vi "CheckRunProbe.vi"(0 "UiDefinition":T1) -> ()   [LabVIEW 2020]
uses:
  UIReferences.ctl
  C:/Users/User/Desktop/Automation/CurrentVersion/LabviewDXFViewer/bin/Release/LabviewDXFViewer.exe
  LabviewDXFViewer/bin/Release/LabviewDXFViewer.exe
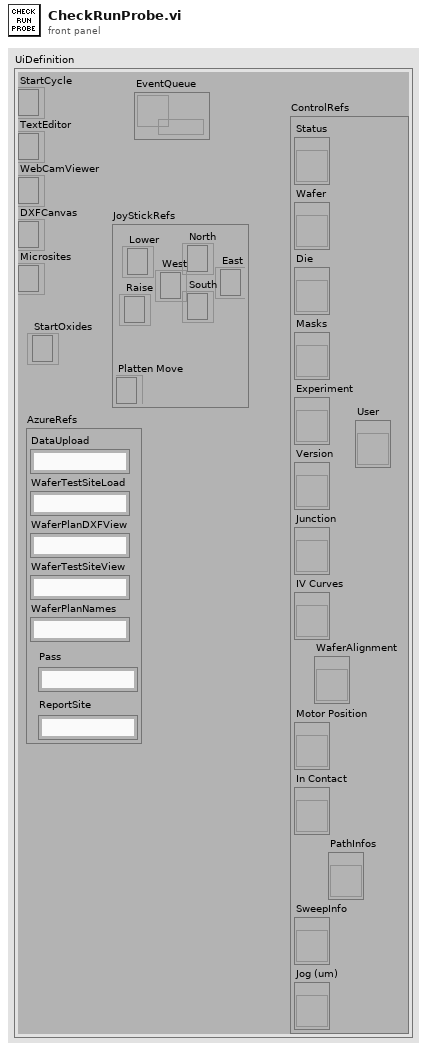
[diagram p1: front panel]
types:
  T1 = typedef "UIReferences.ctl" = cluster{"StartCycle":refnum<k24>, "TextEditor":refnum<k24>, "WebCamViewer":refnum<k24>, "DXFCanvas":refnum<k24>, "Microsites":refnum<k24>, "JoyStickRefs":cluster{"North":refnum<k24>, "Lower":refnum<k24>, "Raise":refnum<k24>, "Platten Move":refnum<k24>, "West":refnum<k24>, "East":refnum<k24>, "South":refnum<k24>}, "AzureRefs":cluster{"DataUpload":string, "WaferTestSiteLoad":string, "WaferPlanDXFView":string, "WaferTestSiteView":string, "WaferPlanNames":string, "Pass":string, "ReportSite":string}, "ControlRefs":cluster{"Status":refnum<vi>, "Wafer":refnum<vi>, "Die":refnum<vi>, "Masks":refnum<vi>, "Experiment":refnum<vi>, "Version":refnum<vi>, "Junction":refnum<vi>, "IV Curves":refnum<vi>, "Motor Position":refnum<vi>, "In Contact":refnum<vi>, "SweepInfo":refnum<vi>, "Jog (um)":refnum<vi>, "PathInfos":refnum<vi>, "User":refnum<vi>, "WaferAlignment":refnum<vi>}, "EventQueue":refnum<queue>, "StartOxides":refnum<k24>}
  T2 = cluster{"Status":refnum<vi>, "Wafer":refnum<vi>, "Die":refnum<vi>, "Masks":refnum<vi>, "Experiment":refnum<vi>, "Version":refnum<vi>, "Junction":refnum<vi>, "IV Curves":refnum<vi>, "Motor Position":refnum<vi>, "In Contact":refnum<vi>, "SweepInfo":refnum<vi>, "Jog (um)":refnum<vi>, "PathInfos":refnum<vi>, "User":refnum<vi>, "WaferAlignment":refnum<vi>}
  T3 = typedef "WaferAlignmentType.ctl" = cluster{"Wafer Units to microns":dbl, "Rotation Misalign":dbl[], "Scale Misalign":dbl, "Steps Per micron":dbl, "Position 1":i32[], "Position 2":i32[], "Lift Distance":i32, "Position 3":i32[], "Jog Height":i32}
  T4 = cluster{"Die":string, "Wafer":string, "Path":path, "url":string, "Experiment":string, "Version":string, "user":string}
  T5 = cluster{"Current Range":dbl, "Source Measure Unit Channel (0: Channel A)":i32, "Waveform":waveform(dbl), "VISA resource name":refnum<visa-resource-name>, "CodeText":string}
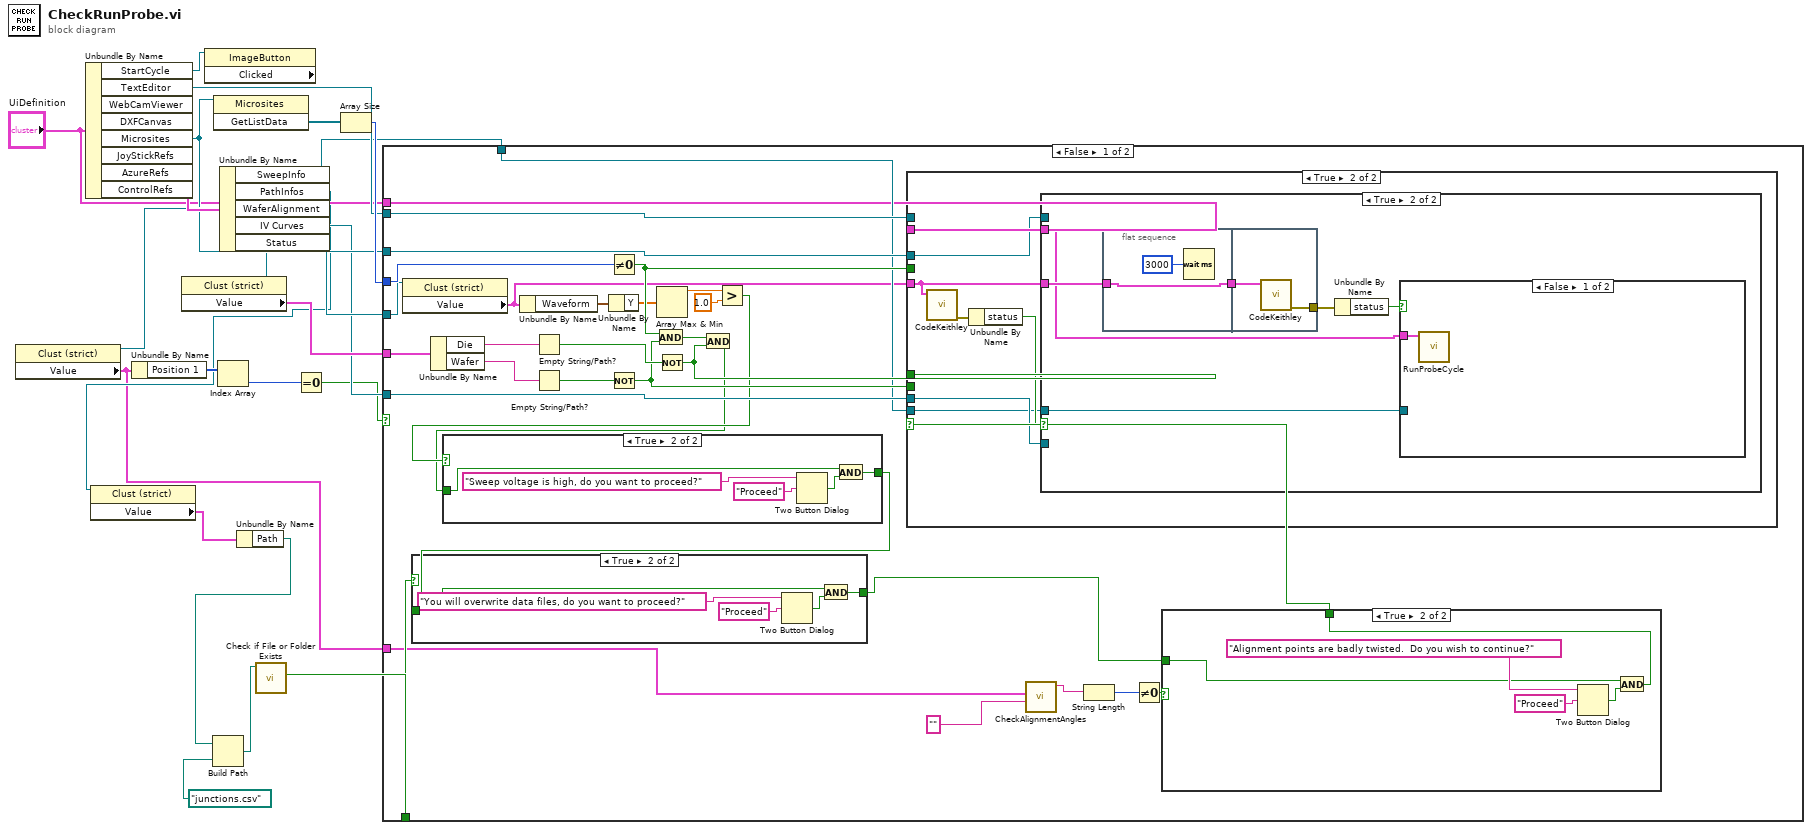
[diagram p0: block diagram]
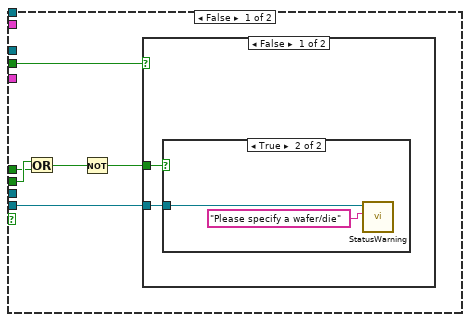
[diagram p5: hidden frame]
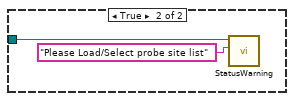
[diagram p7: hidden frame]
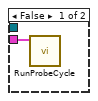
[diagram p8: hidden frame]
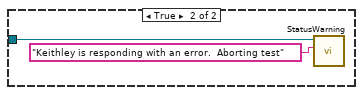
[diagram p9: hidden frame]
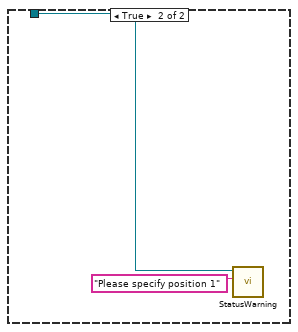
[diagram p10: hidden frame]
diagram:
  n1 = Unbundle By Name("UiDefinition") -> ("StartCycle"=w11:refnum<k24>, "TextEditor"=w15:refnum<k24>, "Microsites"=w16:refnum<k24>, "ControlRefs"=w20:T2)  [unwired: 4 out]
  n2 = property class="ImageButton" props=["Clicked"](reference=w11) -> ()  [unwired: 1 in, 3 out]
  n3 = invoke class="Microsites" method="GetListData"(reference=w16) -> ("GetListData"=w21:refnum<k24>[])  [unwired: 2 in, 2 out]
  n4 = Unbundle By Name(w20) -> ("SweepInfo"=w19:refnum<vi>, "PathInfos"=w7:refnum<vi>, "WaferAlignment"=w17:refnum<vi>, "IV Curves"=w14:refnum<vi>, "Status"=w13:refnum<vi>)
  n5 = property class="Clust (strict)"(reference=w17) -> ("Value"=w1:T3)  [unwired: 1 in, 2 out]
  n6 = property class="Clust (strict)"(reference=w7) -> ("Value"=w6:T4)  [unwired: 1 in, 2 out]
  n7 = Unbundle By Name(w1) -> ("Position 1"=w10:i32[])
  n8 = property class="Clust (strict)"(reference=w7) -> ("Value"=w18:T4)  [unwired: 1 in, 2 out]
  n9 = Index Array(array=w10) -> (element=w9:i32)  [unwired: 1 in]
  n10 = Unbundle By Name(w6) -> ("Path"=w3:path)
  n11 = Build Path(base path=w3, name or relative path=path "junctions.csv") -> (appended path=w4:path)
  n12 = call <vilib>:"Check if File or Folder Exists.vi"("path"=w4) -> ("file or folder exists?"=w2:bool)  [unwired: 8 in, 2 out]
  n13 = Equal To 0?(x=w9) -> (x = 0?=w8:bool)
  n14 = Array Size(array=w21) -> (size(s)=w22:i32)
  n15 = case shown="False" w8 {
    tunnel: w22 -> [w54 _]
    tunnel: w19 -> [w45 _]
    tunnel: w18 -> [w44 _]
    tunnel: w16 -> [w43 _]
    tunnel: w15 -> [w42 _]
    tunnel: w14 -> [w41 _]
    tunnel: w13 -> [w40 w106]
    tunnel: "UiDefinition" -> [w39 _]
    tunnel: w2 -> [w30 _]
    tunnel: w1 -> [w29 _]
    frame False {
      n16 = property class="Clust (strict)"(reference=w45) -> ("Value"=w32:T5)  [unwired: 1 in, 2 out]
      n17 = Unbundle By Name(w44) -> ("Die"=w46:string, "Wafer"=w47:string)
      n18 = Unbundle By Name(w32) -> ("Waveform"=w38:waveform(dbl))
      n19 = Empty String/Path?(string/path=w46) -> (empty?=w50:bool)
      n20 = Empty String/Path?(string/path=w47) -> (empty?=w51:bool)
      n21 = Not Equal To 0?(x=w54) -> (x != 0?=w52:bool)
      n22 = Unbundle By Name(w38) -> ("Y"=w37:dbl[])
      n23 = Not(x=w51) -> (.not. x?=w48:bool)
      n24 = And(x=w52, y=w48) -> (x .and. y?=w53:bool)
      n25 = Array Max & Min(array=w37) -> (max value=w36:dbl)  [unwired: 3 out]
      n26 = Not(x=w50) -> (.not. x?=w49:bool)
      n27 = And(x=w53, y=w49) -> (x .and. y?=w33:bool)
      n28 = Greater?(x=w36, y=1.0) -> (0:w34:bool)
      n29 = case shown="True" w34 {
        tunnel: w33 -> [w67 w68]
        tunnel: [w67 w69] -> w31
        frame False {
        }
        frame True {
          n30 = Two Button Dialog(message="Sweep voltage is high, do you want to proceed?", 2:"Proceed" ("T button name (\"OK\")")) -> (T button?=w70:bool)  [unwired: 1 in]
          n31 = And(x=w68, y=w70) -> (x .and. y?=w69:bool)
        }
      }
      n32 = case shown="True" w30 {
        tunnel: w31 -> [w61 w62]
        tunnel: [w61 w63] -> w24
        frame False {
        }
        frame True {
          n33 = Two Button Dialog(message="You will overwrite data files, do you want to proceed?", 2:"Proceed" ("T button name (\"OK\")")) -> (T button?=w64:bool)  [unwired: 1 in]
          n34 = And(x=w62, y=w64) -> (x .and. y?=w63:bool)
        }
      }
      n35 = call "CheckAlignmentAngles.vi"("Status in"="", "Value"=w29) -> ("Status out"=w27:string)  [unwired: 9 in]
      n36 = String Length(string=w27) -> (length=w26:i32)
      n37 = Not Equal To 0?(x=w26) -> (x != 0?=w25:bool)
      n38 = case shown="True" w25 {
        tunnel: w24 -> [w55 w57]
        tunnel: [w55 w56] -> w23
        frame False {
        }
        frame True {
          n39 = Two Button Dialog(message="Alignment points are badly twisted.  Do you wish to continue?", 2:"Proceed" ("T button name (\"OK\")")) -> (T button?=w58:bool)  [unwired: 1 in]
          n40 = And(x=w57, y=w58) -> (x .and. y?=w56:bool)
        }
      }
      n41 = case shown="True" w23 {
        tunnel: w52 -> [w78 _]
        tunnel: w48 -> [w77 _]
        tunnel: w49 -> [w76 _]
        tunnel: w42 -> [_ _]
        tunnel: w43 -> [_ w91]
        tunnel: w32 -> [_ w85]
        tunnel: w41 -> [_ w90]
        tunnel: w40 -> [w73 w87]
        tunnel: w39 -> [_ w86]
        frame False {
          n42 = Or(x=w77, y=w76) -> (x .or. y?=w75:bool)
          n43 = Not(x=w75) -> (.not. x?=w74:bool)
          n44 = case shown="False" w78 {
            tunnel: w74 -> [w80 _]
            tunnel: w73 -> [w79 w83]
            frame False {
              n45 = case shown="True" w80 {
                tunnel: w79 -> [_ w81]
                frame False {
                }
                frame True {
                  n46 = call "StatusWarning.vi"("Text.Text"="Please specify a wafer/die", "String in"=w81) -> ()  [unwired: 10 in]
                }
              }
            }
            frame True {
              n47 = call "StatusWarning.vi"("Text.Text"="Please Load/Select probe site list", "String in"=w83) -> ()  [unwired: 10 in]
            }
          }
        }
        frame True {
          n48 = call "CodeKeithley.vi"("SweepInfo"=w85) -> ("error out"=w89:errorcluster)  [unwired: 10 in]
          n49 = Unbundle By Name(w89) -> ("status"=w88:bool)
          n50 = case shown="True" w88 {
            tunnel: w91 -> [_ _]
            tunnel: w90 -> [_ _]
            tunnel: w87 -> [_ w98]
            tunnel: w86 -> [w92 w94]
            tunnel: w85 -> [_ w97]
            frame False {
              n51 = call "RunProbeCycle.vi"("UiDefinition"=w92) -> ()  [unwired: 10 in]
            }
            frame True {
              n52 = flat-sequence {
                tunnel: w97 -> [w100]
                tunnel: [w100] -> w93
                tunnel: [w101] -> w96
                tunnel: w93 -> [w102]
                frame #0 {
                  n53 = Wait (ms)(milliseconds to wait=u32 3000) -> ()  [unwired: 1 out]
                }
                frame #1 {
                  n54 = call "CodeKeithley.vi"("SweepInfo"=w102) -> ("error out"=w101:errorcluster)  [unwired: 10 in]
                }
              }
              n55 = Unbundle By Name(w96) -> ("status"=w95:bool)
              n56 = case shown="False" w95 {
                tunnel: w98 -> [_ w104]
                tunnel: w94 -> [w103 _]
                frame False {
                  n57 = call "RunProbeCycle.vi"("UiDefinition"=w103) -> ()  [unwired: 10 in]
                }
                frame True {
                  n58 = call "StatusWarning.vi"("Text.Text"="Keithley is responding with an error.  Aborting test", "String in"=w104) -> ()  [unwired: 10 in]
                }
              }
            }
          }
        }
      }
    }
    frame True {
      n59 = call "StatusWarning.vi"("Text.Text"="Please specify position 1", "String in"=w106) -> ()  [unwired: 10 in]
    }
  }
